vi "LC_Relay_Meas_RAW.vi"(0 "I offset":dbl, 2 "input cluster":T1) -> (3 "VR frequency":dbl, 4 "VL frequency":dbl, 5 "PLL output":cluster{dbl, dbl[], dbl, dbl[]}, 6 "RMS values":dbl[](array[numeric]), 7 "Active Power":dbl[](array[numeric]), 8 "Total power values":dbl[](array[numeric]))   [LabVIEW 2016]
doc: "Calculates RMS, freuquency and power values using raw voltage and current data."
panel:
  out "I RMS":dbl
  out "VR RMS":dbl
  out "VL RMS":dbl
  out "VR phase":dbl[](array[numeric])
  out "VL phase":dbl[](array[numeric])
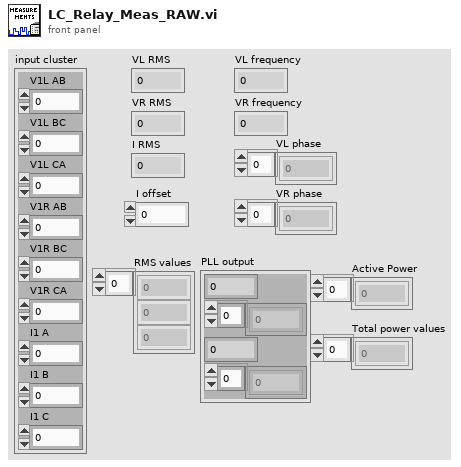
[diagram p1: front panel]
types:
  T1 = cluster{"V1L AB":fxp<+/-,53,11>, "V1L BC":fxp<+/-,53,11>, "V1L CA":fxp<+/-,53,11>, "V1R AB":fxp<+/-,53,11>, "V1R BC":fxp<+/-,53,11>, "V1R CA":fxp<+/-,53,11>, "I1 A":fxp<+/-,53,11>, "I1 B":fxp<+/-,53,11>, "I1 C":fxp<+/-,53,11>}
  T2 = cluster{"V1L AB":fxp<+/-,53,11>, "V1L BC":fxp<+/-,53,11>, "V1L CA":fxp<+/-,53,11>}
  T3 = cluster{"V1R AB":fxp<+/-,53,11>, "V1R BC":fxp<+/-,53,11>, "V1R CA":fxp<+/-,53,11>}
  T4 = cluster{"I1 A":fxp<+/-,53,11>, "I1 B":fxp<+/-,53,11>, "I1 C":fxp<+/-,53,11>}
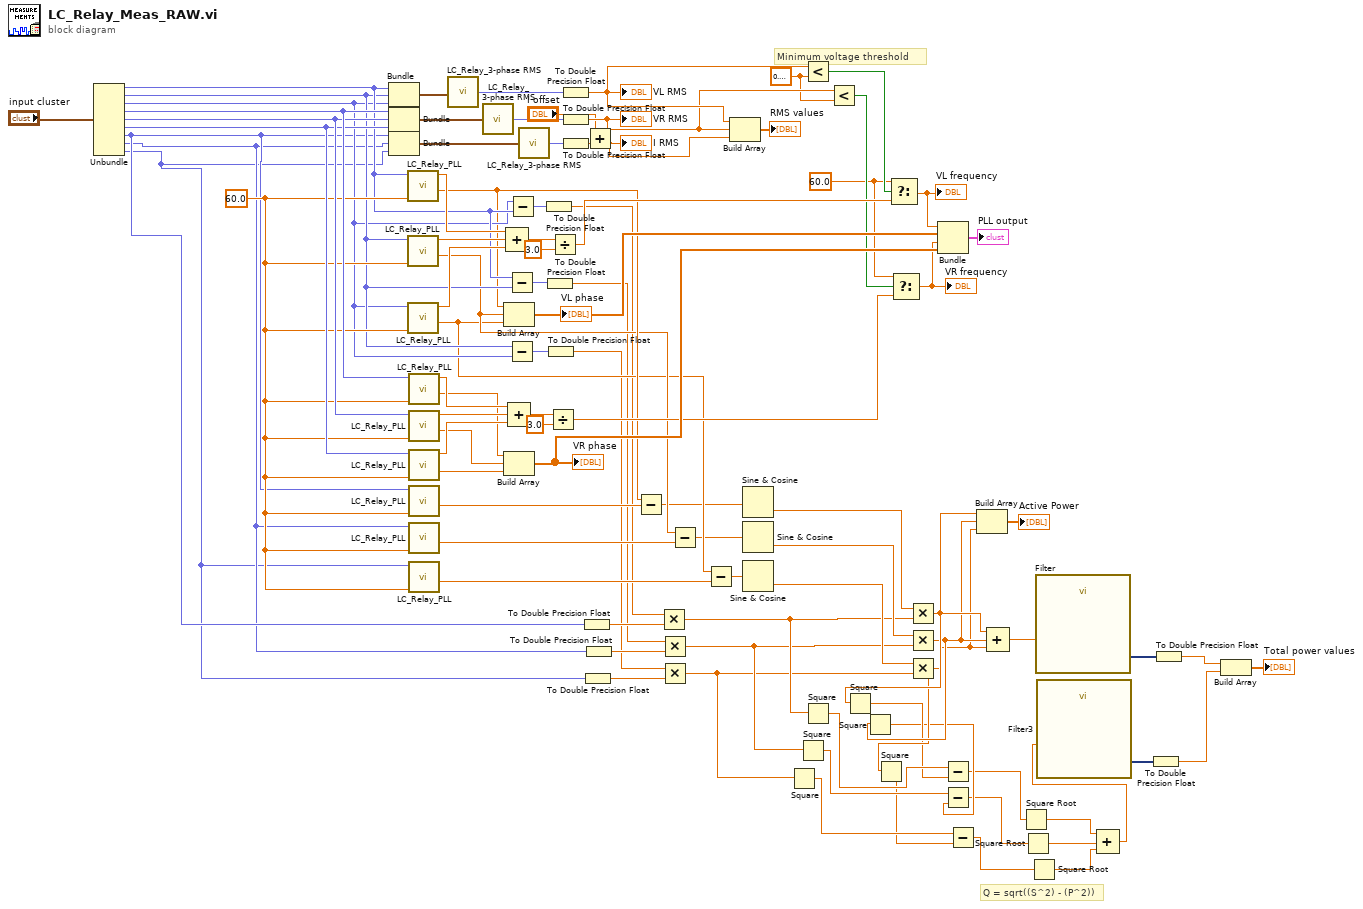
[diagram p0: block diagram]
diagram:
  w54 = 60.0 ("t")
  w58 = 0.30000001192092896 ("y")
  w87 = 60.0 ("fc")
  # "Q = sqrt((S^2) - (P^2))"
  # "Minimum voltage threshold"
  n1 = Unbundle("input cluster") -> ("V1L AB"=w66:fxp<+/-,53,11>, "V1L BC"=w65:fxp<+/-,53,11>, "V1L CA"=w64:fxp<+/-,53,11>, "V1R AB"=w93:fxp<+/-,53,11>, "V1R BC"=w92:fxp<+/-,53,11>, "V1R CA"=w91:fxp<+/-,53,11>, "I1 A"=w40:fxp<+/-,53,11>, "I1 B"=w36:fxp<+/-,53,11>, "I1 C"=w33:fxp<+/-,53,11>)
  n2 = Bundle("V1L AB"=w66, "V1L BC"=w65, "V1L CA"=w64) -> (w73:T2)  [unwired: 1 in]
  n3 = Bundle("V1R AB"=w93, "V1R BC"=w92, "V1R CA"=w91) -> (w72:T3)  [unwired: 1 in]
  n4 = Bundle("I1 A"=w40, "I1 B"=w36, "I1 C"=w33) -> (w71:T4)  [unwired: 1 in]
  n5 = call "LC_Relay_PLL.vi"("fc"=w87, "input"=w66) -> ("phase"=w50:dbl, "frequency"=w86:dbl)  [unwired: 8 in]
  n6 = call "LC_Relay_PLL.vi"("fc"=w87, "input"=w65) -> ("phase"=w48:dbl, "frequency"=w85:dbl)  [unwired: 8 in]
  n7 = call "LC_Relay_PLL.vi"("fc"=w87, "input"=w64) -> ("phase"=w46:dbl, "frequency"=w84:dbl)  [unwired: 8 in]
  n8 = call "LC_Relay_PLL.vi"("fc"=w87, "input"=w93) -> ("phase"=w76:dbl, "frequency"=w82:dbl)  [unwired: 8 in]
  n9 = call "LC_Relay_PLL.vi"("fc"=w87, "input"=w92) -> ("phase"=w75:dbl, "frequency"=w83:dbl)  [unwired: 8 in]
  n10 = call "LC_Relay_PLL.vi"("fc"=w87, "input"=w91) -> ("phase"=w74:dbl, "frequency"=w81:dbl)  [unwired: 8 in]
  n11 = call "LC_Relay_PLL.vi"("fc"=w87, "input"=w40) -> ("phase"=w49:dbl)  [unwired: 8 in, 1 out]
  n12 = call "LC_Relay_PLL.vi"("fc"=w87, "input"=w36) -> ("phase"=w47:dbl)  [unwired: 8 in, 1 out]
  n13 = call "LC_Relay_PLL.vi"("fc"=w87, "input"=w33) -> ("phase"=w45:dbl)  [unwired: 8 in, 1 out]
  n14 = call "LC_Relay_3-phase RMS.vi"("Vabc"=w73) -> ("RMS"=w63:fxp<+,55,5>)  [unwired: 4 in]
  n15 = call "LC_Relay_3-phase RMS.vi"("Vabc"=w72) -> ("RMS"=w62:fxp<+,55,5>)  [unwired: 4 in]
  n16 = Build Array(w50, w48, w46) -> (w69:dbl[])
  "VL phase" <- w69
  n17 = Build Array(w76, w75, w74) -> (w68:dbl[])
  "VR phase" <- w68
  n18 = Compound Arithmetic op=ADD(w86, w85, w84) -> (w80:dbl)
  n19 = Subtract(x=w66, y=w65) -> (x-y=w89:fxp<+/-,53,11>)
  n20 = Subtract(x=w65, y=w64) -> (x-y=w88:fxp<+/-,53,11>)
  n21 = Subtract(x=w64, y=w66) -> (x-y=w90:fxp<+/-,53,11>)
  n22 = Compound Arithmetic op=ADD(w82, w83, w81) -> (w77:dbl)
  n23 = call "LC_Relay_3-phase RMS.vi"("Vabc"=w71) -> ("RMS"=w70:fxp<+,55,5>)  [unwired: 4 in]
  n24 = To Double Precision Float(number=w90) -> (double precision float=w41:dbl)
  n25 = To Double Precision Float(number=w89) -> (double precision float=w38:dbl)
  n26 = To Double Precision Float(number=w88) -> (double precision float=w35:dbl)
  n27 = Divide(x=w77, y=3.0) -> (x/y=w53:dbl)
  n28 = Divide(x=w80, y=3.0) -> (x/y=w56:dbl)
  n29 = To Double Precision Float(number=w63) -> (double precision float=w61:dbl)
  "VL RMS" <- w61
  n30 = To Double Precision Float(number=w62) -> (double precision float=w60:dbl)
  "VR RMS" <- w60
  n31 = To Double Precision Float(number=w70) -> (double precision float=w59:dbl)
  n32 = To Double Precision Float(number=w40) -> (double precision float=w39:dbl)
  n33 = To Double Precision Float(number=w33) -> (double precision float=w34:dbl)
  n34 = To Double Precision Float(number=w36) -> (double precision float=w37:dbl)
  n35 = Add(x="I offset", y=w59) -> (x+y=w2:dbl)
  "I RMS" <- w2
  n36 = Subtract(x=w50, y=w49) -> (x-y=w44:dbl)
  n37 = Multiply(x=w41, y=w39) -> (x*y=w21:dbl)
  n38 = Multiply(x=w38, y=w37) -> (x*y=w20:dbl)
  n39 = Multiply(x=w35, y=w34) -> (x*y=w19:dbl)
  n40 = Subtract(x=w48, y=w47) -> (x-y=w43:dbl)
  n41 = Subtract(x=w46, y=w45) -> (x-y=w42:dbl)
  n42 = Build Array(w61, w60, w2) -> (→"RMS values":dbl[])
  n43 = Sine & Cosine(0:w44) -> (2:w32:dbl)  [unwired: 1 out]
  n44 = Sine & Cosine(0:w43) -> (2:w31:dbl)  [unwired: 1 out]
  n45 = Sine & Cosine(0:w42) -> (2:w30:dbl)  [unwired: 1 out]
  n46 = Square(x=w19) -> (x^2=w11:dbl)
  n47 = Square(x=w20) -> (x^2=w13:dbl)
  n48 = Less?(x=w61, y=w58) -> (x < y?=w57:bool)
  n49 = Square(x=w21) -> (x^2=w15:dbl)
  n50 = Less?(x=w60, y=w58) -> (x < y?=w55:bool)
  n51 = Select(t=w54, s=w57, f=w56) -> (s? t:f=w52:dbl)
  "VL frequency" <- w52
  n52 = Select(t=w54, s=w55, f=w53) -> (s? t:f=w51:dbl)
  "VR frequency" <- w51
  n53 = Multiply(x=w32, y=w21) -> (x*y=w18:dbl)
  n54 = Square(x=w18) -> (x^2=w14:dbl)
  n55 = Multiply(x=w31, y=w20) -> (x*y=w17:dbl)
  n56 = Square(x=w17) -> (x^2=w12:dbl)
  n57 = Multiply(x=w30, y=w19) -> (x*y=w16:dbl)
  n58 = Square(x=w16) -> (x^2=w10:dbl)
  n59 = Bundle("t"=w52, w69, "t"=w51, w68) -> (→"PLL output":cluster{"t":dbl, dbl[], "t":dbl, dbl[]})  [unwired: 1 in]
  n60 = Subtract(x=w15, y=w14) -> (x-y=w9:dbl)
  n61 = Subtract(x=w13, y=w12) -> (x-y=w8:dbl)
  n62 = Subtract(x=w11, y=w10) -> (x-y=w7:dbl)
  n63 = Build Array(w18, w17, w16) -> (→"Active Power":dbl[])
  n64 = Compound Arithmetic op=ADD(w18, w17, w16) -> (w29:dbl)
  n65 = Square Root(x=w9) -> (sqrt(x)=w6:dbl)
  n66 = Square Root(x=w8) -> (sqrt(x)=w5:dbl)
  n67 = Square Root(x=w7) -> (sqrt(x)=w4:dbl)
  n68 = call "Filter"("Signal"=w29) -> ("Filtered Signal"=w26:dynamicdata)  [unwired: 9 in, 1 out]
  n69 = Compound Arithmetic op=ADD(w6, w5, w4) -> (w3:dbl)
  n70 = call "Filter3"("Signal"=w3) -> ("Filtered Signal"=w28:dynamicdata)  [unwired: 9 in, 1 out]
  n71 = To Double Precision Float(number=w28) -> (double precision float=w24:dbl)
  n72 = To Double Precision Float(number=w26) -> (double precision float=w25:dbl)
  n73 = Build Array(w25, w24) -> (→"Total power values":dbl[])
